vi "Take Area Image.vi"(6 "Image Name":string="composite image", 7 "Quality":enum16{"perfect", "medium", "low"}(ring), 8 "error in":errorcluster, 9 "Field of View":cluster{"Size-X(mm)":dbl, "Size-Y(mm)":dbl}, 10 "Image Center":refnum<class "Vec3d Class.lvclass">, 11 "CameraTool in":refnum<class "CameraTool Class.lvclass">) -> (0 "error out":errorcluster, 2 "Physical Image":T1, 3 "CameraTool out":refnum<class "CameraTool Class.lvclass">)   [LabVIEW 2011, in "CameraTool Class.lvclass"]
uses:
  CameraTool Class.lvclass
  Utils/Type Definitions/Physical Image.ctl
  Vec3d Class/Vec3d Class.lvclass
  <vilib>/vision/Image Controls.llb/IMAQ Image.ctl
  Config Manager Class/Type Definitions/Camera Enum.ctl
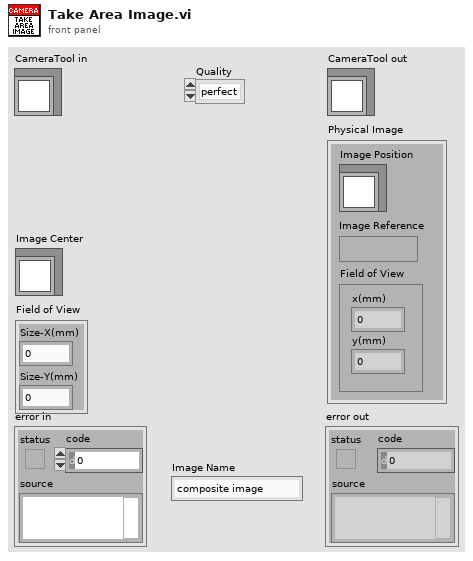
[diagram p1: front panel]
types:
  T1 = typedef "Physical Image.ctl" = cluster{"Image Position":refnum<class "Vec3d Class.lvclass">, "Image Reference":T2, "Field of View":cluster{"x(mm)":dbl, "y(mm)":dbl}}
  T2 = typedef "IMAQ Image.ctl" = refnum<image>
  T3 = typedef "Camera Enum.ctl" = enum16{"GANTRY HEAD", "NEEDLE CALIBRATION X", "NEEDLE CALIBRATION Y"}
  T4 = typedef "Gantry_Camera.ctl" = cluster{"IMAQ Session":T5, "Group":u32, "Open?":bool, "Interface Name":string, "Field of View":cluster{"x-mm":dbl, "y-mm":dbl}, "Name":T3}
  T5 = typedef "IMAQdx.ctl" = refnum<k21>
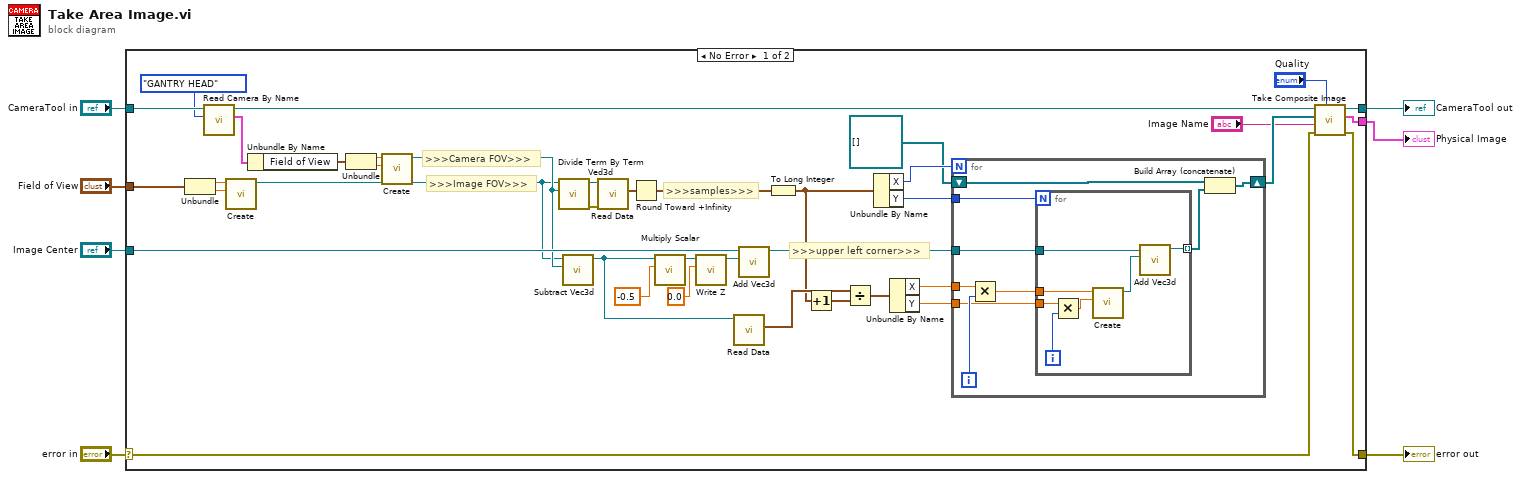
[diagram p0: block diagram]
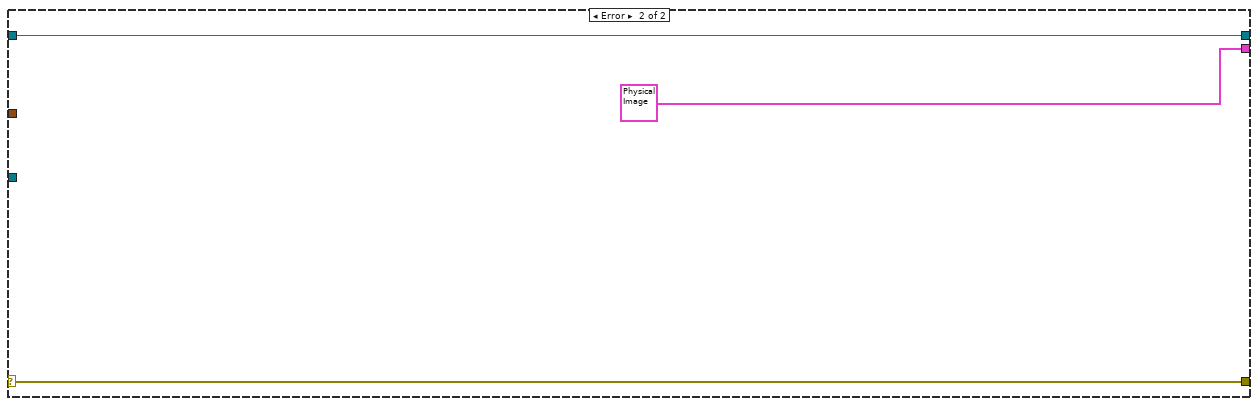
[diagram p2: hidden frame]
diagram:
  n1 = case shown="No Error" "error in" {
    selector: "error in" -> [w17 w65]
    tunnel: [w16 w65] -> w6
    tunnel: [w26 w64] -> w4
    tunnel: "CameraTool in" -> [w46 w64]
    tunnel: "Field of View" -> [w44 _]
    tunnel: "Image Center" -> [w36 _]
    tunnel: [w15 T1 {"Image Position"=refnum, "Image Reference"=refnum, "Field of View"={"x(mm)"=0.0, "y(mm)"=0.0}} ("Physical Image")] -> w1
    frame No Error {
      # ">>>upper left corner>>>"
      # ">>>samples>>>"
      # ">>>Camera FOV>>>"
      # ">>>Image FOV>>>"
      n2 = Unbundle(w44) -> ("Size-X(mm)"=w43:dbl, "Size-Y(mm)"=w42:dbl)
      n3 = call-dynamic "Read Camera By Name.vi"("Camera Name"=Camera_Enum."GANTRY HEAD", "Gantry in"=w46) -> ("Camera"=w45:T4, "Gantry out"=w27:refnum<class "CameraTool Class.lvclass">)  [unwired: 7 in, 1 out]
      n4 = call "Create.vi"("Y"=w42, "X"=w43) -> ("Vec3d Class out"=w9:refnum<class "Vec3d Class.lvclass">)  [unwired: 8 in, 1 out]
      n5 = Unbundle By Name(w45) -> ("Field of View"=w39:cluster{"x-mm":dbl, "y-mm":dbl})
      n6 = Unbundle(w39) -> ("x-mm"=w41:dbl, "y-mm"=w40:dbl)
      n7 = call "Create.vi"("Y"=w40, "X"=w41) -> ("Vec3d Class out"=w10:refnum<class "Vec3d Class.lvclass">)  [unwired: 8 in, 1 out]
      n8 = call-dynamic "Divide Term By Term Ved3d.vi"("Vec3d in 2"=w10, "Vec3d in 1"=w9) -> ("error out"=w38:errorcluster, "Vec3d Class out"=w37:refnum<class "Vec3d Class.lvclass">)  [unwired: 8 in]
      n9 = call "Subtract Vec3d.vi"("Vec3d in 2"=w10, "Vec3d in 1"=w9) -> ("Vec3d Class out"=w31:refnum<class "Vec3d Class.lvclass">)  [unwired: 8 in, 1 out]
      n10 = call-dynamic "Read Data.vi"("error in (no error)"=w38, "Vec3d Class in"=w37) -> ("Data"=w12:cluster{"X":dbl, "Y":dbl, "Z":dbl})  [unwired: 7 in, 2 out]
      n11 = Round Toward +Infinity(x=w12) -> (ceil(x): smallest int >= x=w11:cluster{"X":dbl, "Y":dbl, "Z":dbl})
      n12 = call-dynamic "Multiply Scalar.vi"("Scale"=-0.5, "Vec3d in"=w31) -> ("Vec3d out"=w34:refnum<class "Vec3d Class.lvclass">)  [unwired: 8 in, 1 out]
      n13 = call-dynamic "Write Z.vi"("Z"=0.0, "Vec3d Class in"=w34) -> ("Vec3d Class out"=w32:refnum<class "Vec3d Class.lvclass">)  [unwired: 8 in, 1 out]
      n14 = call-dynamic "Read Data.vi"("Vec3d Class in"=w31) -> ("Data"=w29:cluster{"X":dbl, "Y":dbl, "Z":dbl})  [unwired: 8 in, 2 out]
      n15 = call-dynamic "Add Vec3d.vi"(10:"Vec3d Class in"=w32, 11:"Vec3d Class in"=w36) -> ("Vec3d Class out"=w22:refnum<class "Vec3d Class.lvclass">)  [unwired: 8 in, 1 out]
      n16 = To Long Integer(number=w11) -> (32bit integer=w24:cluster{"X":i32, "Y":i32, "Z":i32})
      n17 = Increment(x=w24) -> (x+1=w30:cluster{"X":i32, "Y":i32, "Z":i32})
      n18 = Divide(x=w29, y=w30) -> (x/y=w28:cluster{"X":dbl, "Y":dbl, "Z":dbl})
      n19 = Unbundle By Name(w24) -> ("X"=w25:i32, "Y"=w23:i32)
      n20 = Unbundle By Name(w28) -> ("X"=w21:dbl, "Y"=w20:dbl)
      n21 = for {
        N: w25 -> [_]
        tunnel: w23 -> [w55]
        tunnel: w22 -> [w54]
        tunnel: w21 -> [w52]
        tunnel: w20 -> [w51]
        shift-right: [w47] -> w18
        shift-left: refnum<class "Vec3d Class.lvclass">[] [] -> [w48]
        i -> [w53]
        n22 = Multiply(x=w52, y=w53) -> (x*y=w50:dbl)
        n23 = for {
          N: w55 -> [_]
          tunnel: w54 -> [w57]
          tunnel: w51 -> [w62]
          tunnel: w50 -> [w59]
          tunnel: [w56] -> w49 mode=indexing
          i -> [w61]
          n24 = Multiply(x=w62, y=w61) -> (x*y=w60:dbl)
          n25 = call "Create.vi"("Y"=w60, "X"=w59) -> ("Vec3d Class out"=w58:refnum<class "Vec3d Class.lvclass">)  [unwired: 8 in, 1 out]
          n26 = call-dynamic "Add Vec3d.vi"(10:"Vec3d Class in"=w58, 11:"Vec3d Class in"=w57) -> ("Vec3d Class out"=w56:refnum<class "Vec3d Class.lvclass">)  [unwired: 8 in, 1 out]
        }
        n27 = Build Array (concatenate)(w48, w49) -> (w47:refnum<class "Vec3d Class.lvclass">[])
      }
      n28 = call "Take Composite Image.vi"("Quality"="Quality", "error in"=w17, "Image Name"="Image Name", "Points"=w18, "CameraTool in"=w27) -> ("error out"=w16:errorcluster, "Physical Image"=w15:T1, "CameraTool out"=w26:refnum<class "CameraTool Class.lvclass">)  [unwired: 4 in]
    }
    frame Error {
    }
  }
  "error out" <- w6
  "CameraTool out" <- w4
  "Physical Image" <- w1
